vi "NIDmm T12.vi"(8 "error in (no error)":errorcluster, 9 "Range (Amps)":dbl, 10 "Resolution in Digits":dbl, 11 "IVI Refnum in":refnum<k15>) -> (0 "error out":errorcluster, 2 "Over Range?":bool, 3 "Measurement":dbl)   [LabVIEW 2021]
uses:
  <instrlib>/niDMM/nidmm.llb/niDMM Function.ctl
  <instrlib>/niDMM/nidmm.llb/niDMM Configure Measurement Digits.vi
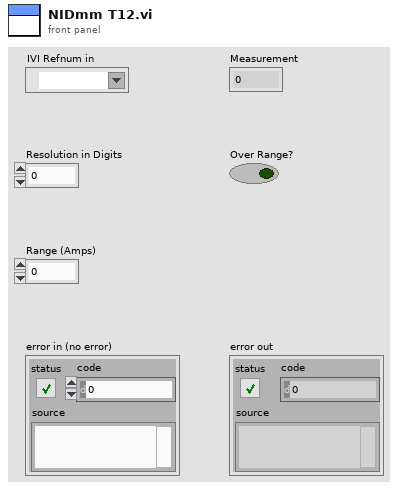
[diagram p1: front panel]
types:
  T1 = typedef "niDMM Function.ctl" = enum16{"DC Volts", "AC Volts", "DC Current", "AC Current", "2-wire Resistance", "4-wire Resistance", "Diode", "Frequency", "Period", "AC Volts DC Coupled", "Capacitance", "Inductance", "Temperature"}
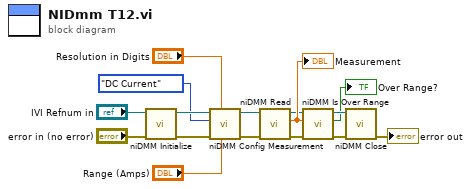
[diagram p0: block diagram]
diagram:
  n1 = call <instrlib>:"niDMM Initialize.vi"("error in (no error)"="error in (no error)", "Instrument Descriptor"="IVI Refnum in") -> ("error out"=w14:errorcluster, "instrument handle out"=w12:refnum<k15>)  [unwired: 8 in]
  n2 = call-poly <instrlib>:"niDMM Config Measurement.vi"("Range"="Range (Amps)", "Resolution in Digits"="Resolution in Digits", "error in (no error)"=w14, "Function"=niDMM_Function."DC Current", "instrument handle"=w12) -> ("error out"=w2:errorcluster, "instrument handle out"=w3:refnum<k15>)  [unwired: 5 in]
  n3 = call <instrlib>:"niDMM Read.vi"("error in (no error)"=w2, "instrument handle"=w3) -> ("error out"=w5:errorcluster, "Measurement"=w10:dbl, "instrument handle out"=w4:refnum<k15>)  [unwired: 7 in]
  "Measurement" <- w10
  n4 = call <instrlib>:"niDMM Is Over Range.vi"("error in (no error)"=w5, "Measurement"=w10, "instrument handle"=w4) -> ("error out"=w6:errorcluster, "Over Range?"=→"Over Range?":bool, "instrument handle out"=w16:refnum<k15>)  [unwired: 6 in]
  n5 = call <instrlib>:"niDMM Close.vi"("error in (no error)"=w6, "instrument handle"=w16) -> ("error out"=→"error out":errorcluster)  [unwired: 9 in]
